vi "Filter.vi"(8 "error in":errorcluster, 9 "Image original":T1, 10 "Image copy":T1, 11 "Session Config":T2) -> (0 "error out":errorcluster, 1 "Session Out":T2, 2 "Data":string, 3 "Image Out":T1)   [LabVIEW 2020]
uses:
  <vilib>/userDefined/High Color/IMAQdx.ctl
  <vilib>/vision/Image Controls.llb/IMAQ Image.ctl
  <vilib>/vision/NI_Vision_Development_Module.lvlib
  <vilib>/vision/driver/NI_Vision_Acquisition_Software.lvlib
panel:
  out "Image":T1(plugin-control)
  out "Found?":bool
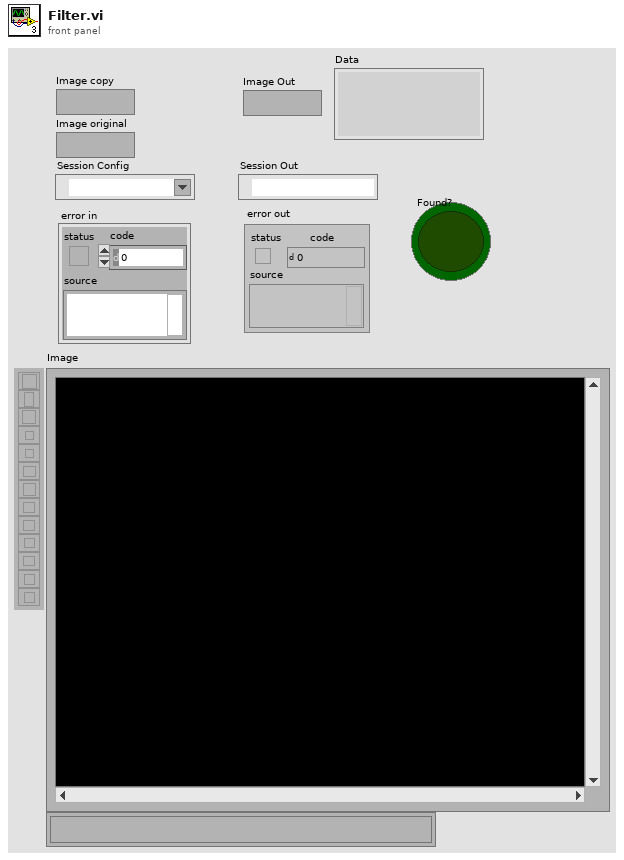
[diagram p1: front panel]
types:
  T1 = typedef "IMAQ Image.ctl" = refnum<image>
  T2 = typedef "IMAQdx.ctl" = refnum<k21>
  T3 = typedef "QR Code Report.ctl" = cluster{"Found?":bool, "Data":string, "Bounding Box":cluster{"x":sgl, "y":sgl}[], "Errors Corrected":u32, "Dimensions (Rows/Cols)":u32, "Version":u32, "QR Model":T4, "Stream Mode":T5, "Barcode Polarity":T6, "Mirrored?":bool, "Append Stream Position":u32, "Size of Append Stream":u32, "First EAN-128 ID":i32, "First Alternate Language ID":i32, "Append Stream ID":u32, "Minimum Edge Strength":u32, "Demodulation Mode":T7, "Cell Sample Size":T8, "Cell Filter Mode":T9}
  T4 = typedef "QR Code Model Type.ctl" = i32
  T5 = typedef "QR Code Stream Mode Type.ctl" = i32
  T6 = typedef "Data Matrix Polarity.ctl" = i32
  T7 = typedef "Demodulation Mode.ctl" = i32
  T8 = typedef "Cell Sample Size.ctl" = i32
  T9 = typedef "Cell Filter Mode.ctl" = i32
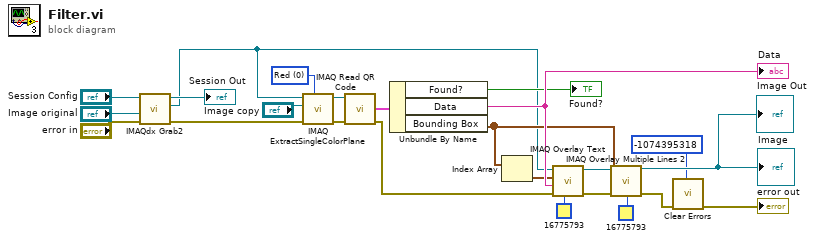
[diagram p0: block diagram]
diagram:
  w9 = 0 items=["Red", "Green", "Blue", "Hue", "Saturation", "Luminance", "Value", "Intensity"] ("Color Plane")
  n1 = call <vilib>:"IMAQdx Grab2.vi"("error in"="error in", "Image In"="Image original", "Session In"="Session Config") -> ("error out"=w1:errorcluster, "Image Out"=w2:T1, "Session Out"=→"Session Out":T2)  [unwired: 5 in, 1 out]
  n2 = call "IMAQ ExtractSingleColorPlane"("Color Plane"=w9, "error in (no error)"=w1, "Image Dst"="Image copy", "Image Src"=w2) -> ("error out"=w13:errorcluster, "Image Dst Out"=w20:T1)  [unwired: 6 in]
  n3 = call "IMAQ Read QR Code"("error in (no error)"=w13, "Image"=w20) -> ("error out"=w18:errorcluster, "QR Code Report"=w14:T3)  [unwired: 6 in, 2 out]
  n4 = Unbundle By Name(w14) -> ("Found?"=→"Found?":bool, "Data"=w23:string, "Bounding Box"=w17:cluster{"x":sgl, "y":sgl}[])
  "Data" <- w23
  n5 = Index Array(array=w17) -> (element=w16:cluster{"x":sgl, "y":sgl})  [unwired: 1 in]
  n6 = call "IMAQ Overlay Text"("Text Color (black)"=u32 16775793, "error in (no error)"=w18, "String"=w23, "Origin"=w16, "Image"=w2) -> ("error out"=w7:errorcluster, "Image Out"=w19:T1)  [unwired: 5 in]
  n7 = call "IMAQ Overlay Multiple Lines 2"("Image"=w19, "Line End Points"=w17, "Color"=u32 16775793, "error in (no error)"=w7) -> ("Image Out"=→"Image" →"Image Out":T1, "error out"=w21:errorcluster)  [unwired: 10 in]
  n8 = call <vilib>:"Clear Errors.vi"("error in (no error)"=w21, "specific error code to clear (0: all)"=-1074395318) -> ("error out"=→"error out":errorcluster)  [unwired: 4 in, 1 out]
